vi "Update Enum Value.vi"(9 "Value":string, 10 "Tree Tag":string, 11 "UI Data In":refnum<class "Settings UI.lvclass">) -> (3 "UI Data Out":refnum<class "Settings UI.lvclass">)   [LabVIEW 2024, in "Output Sequencer.lvlib" / "Settings UI.lvclass"]
uses:
  Settings UI.lvclass
  Settings UI.lvclass/Settings UI.ctl
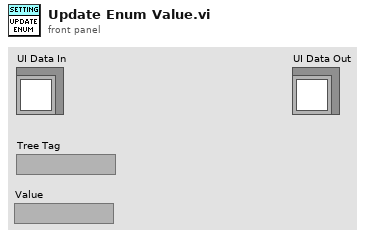
[diagram p1: front panel]
types:
  T1 = typedef "Output Sequencer.lvlib/Settings UI.lvclass/Tree Index Enum.ctl" = enum16{"General Settings", "Num Steps", "Num Analog", "Num Digital", "Show Confirmation", "Interp Priority", "Adv Timing", "Enable Conditions", "Seq Execution", "Reset Test Start", "Only When Test", "Delay After Test", "Start condition", "Re-triggering", "Stop condition", "Stop After Cycles", "Stop Values", "Default Values", "Default Analog", "Default Digital", "Steps", "Step #", "Description", "Precondition", "Duration", "Mode", "Delay Between Vals", "Analog Values", "Digital Values", "Postcondition", "On True", "On False"}
  T2 = typedef "Output Sequencer.lvlib/Settings UI.lvclass/Tree Item Settings.ctl" = cluster{"Tree Label":string, "Indent Level":i32, "Data Type":T3, "Numeric Range":cluster{"Min":dbl, "Max":dbl, "Inc":dbl}, "Allowed Values":string[], "Default Value":string, "Description":string}
  T3 = typedef "Output Sequencer.lvlib/Settings UI.lvclass/Data Type.ctl" = i16
  T4 = typedef "Output Sequencer.lvlib/Settings UI.lvclass/Step Settings.ctl" = cluster{"Description":string, "Precondition":string, "Duration":dbl, "Mode":string, "Delay Between Values":dbl, "Analog Values":string[], "Digital Values":string[], "Postcondition":string, "On True":string, "On False":string}
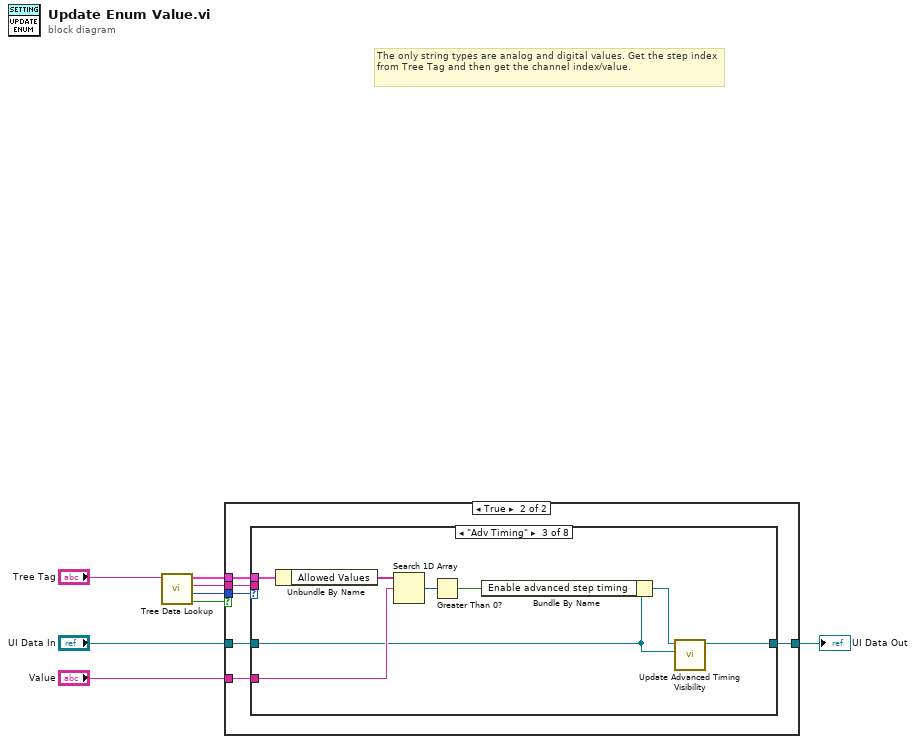
[diagram p0: block diagram]
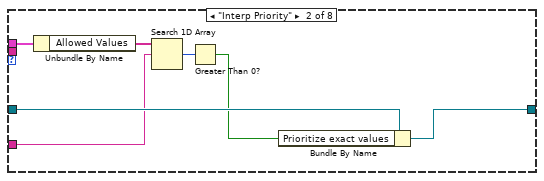
[diagram p4: hidden frame]
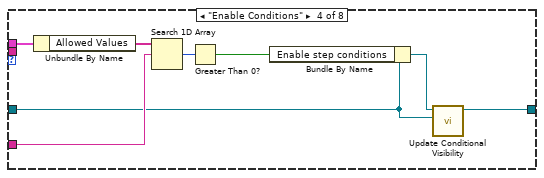
[diagram p5: hidden frame]
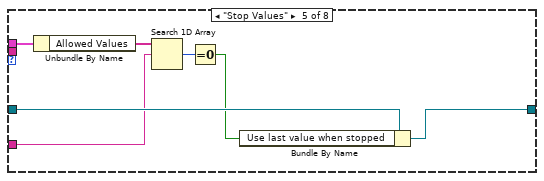
[diagram p6: hidden frame]
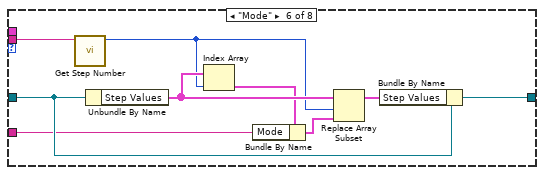
[diagram p7: hidden frame]
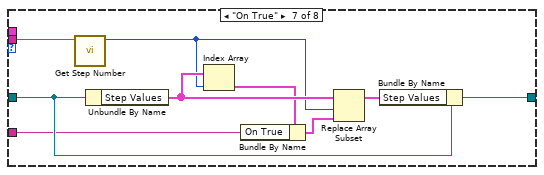
[diagram p8: hidden frame]
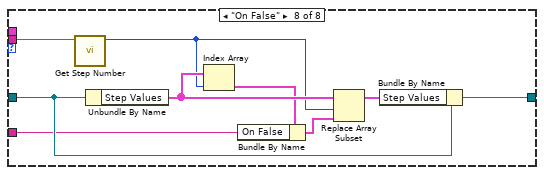
[diagram p9: hidden frame]
diagram:
  # "The only string types are analog and digital values. Get the step index from Tree Tag and then get the channel index/value."
  n1 = call "Tree Data Lookup.vi"("Tag in"="Tree Tag") -> ("Found?"=w4:bool, "Tree Index Enum"=w3:T1, "Tag out"=w1:string, "Tree Data"=w2:T2)  [unwired: 5 in, 2 out]
  n2 = case shown="True" w4 {
    tunnel: "UI Data In" -> [w9 w15]
    tunnel: [w9 w14] -> w7
    tunnel: "Value" -> [_ w13]
    tunnel: w3 -> [_ w12]
    tunnel: w2 -> [_ w11]
    tunnel: w1 -> [_ w10]
    frame False {
    }
    frame True {
      n3 = case shown="\"Adv Timing\"" w12 {
        tunnel: w15 -> [w16 w23 w27 w35 w46 w51 w60 w69]
        tunnel: [w16 w18 w24 w32 w41 w50 w59 w68] -> w14
        tunnel: w13 -> [_ w21 w30 w38 w44 w49 w58 w67]
        tunnel: w11 -> [_ w17 w26 w34 w40 _ _ _]
        tunnel: w10 -> [_ _ _ _ _ w48 w57 w66]
        frame Default {
        }
        frame "Interp Priority" {
          n4 = Unbundle By Name(w17) -> ("Allowed Values"=w22:string[])
          n5 = Search 1D Array(1D array=w22, element=w21) -> (index of element=w20:i32)  [unwired: 1 in]
          n6 = Greater Than 0?(x=w20) -> (x > 0?=w19:bool)
          n7 = Bundle By Name(cluster=w23, "Prioritize exact values"=w19) -> (w18:refnum<class "Settings UI.lvclass">)
        }
        frame "Adv Timing" {
          n8 = Unbundle By Name(w26) -> ("Allowed Values"=w31:string[])
          n9 = Search 1D Array(1D array=w31, element=w30) -> (index of element=w29:i32)  [unwired: 1 in]
          n10 = Greater Than 0?(x=w29) -> (x > 0?=w28:bool)
          n11 = Bundle By Name(cluster=w27, "Enable advanced step timing"=w28) -> (w25:refnum<class "Settings UI.lvclass">)
          n12 = call "Update Advanced Timing Visibility.vi"("Previous UI Data in"=w27, "New UI Data in"=w25) -> ("New UI Data out"=w24:refnum<class "Settings UI.lvclass">)  [unwired: 8 in, 1 out]
        }
        frame "Enable Conditions" {
          n13 = Unbundle By Name(w34) -> ("Allowed Values"=w39:string[])
          n14 = Search 1D Array(1D array=w39, element=w38) -> (index of element=w37:i32)  [unwired: 1 in]
          n15 = Greater Than 0?(x=w37) -> (x > 0?=w36:bool)
          n16 = Bundle By Name(cluster=w35, "Enable step conditions"=w36) -> (w33:refnum<class "Settings UI.lvclass">)
          n17 = call "Update Conditional Visibility.vi"("Previous UI Data in"=w35, "New UI Data in"=w33) -> ("New UI Data out"=w32:refnum<class "Settings UI.lvclass">)  [unwired: 9 in]
        }
        frame "Stop Values" {
          n18 = Unbundle By Name(w40) -> ("Allowed Values"=w45:string[])
          n19 = Search 1D Array(1D array=w45, element=w44) -> (index of element=w43:i32)  [unwired: 1 in]
          n20 = Equal To 0?(x=w43) -> (x = 0?=w42:bool)
          n21 = Bundle By Name(cluster=w46, "Use last value when stopped"=w42) -> (w41:refnum<class "Settings UI.lvclass">)
        }
        frame "Mode" {
          n22 = call "Get Step Number.vi"("Tree Tag"=w48) -> ("Step Number"=w47:i32)  [unwired: 8 in, 2 out]
          n23 = Unbundle By Name(w51) -> ("Step Values"=w55:T4[])
          n24 = Index Array(array=w55, index=w47) -> (element=w53:T4)
          n25 = Bundle By Name(cluster=w53, "Mode"=w49) -> (w52:T4)
          n26 = Replace Array Subset(array=w55, new element=w52, index=w47) -> (w54:T4[])
          n27 = Bundle By Name(cluster=w51, "Step Values"=w54) -> (w50:refnum<class "Settings UI.lvclass">)
        }
        frame "On True" {
          n28 = call "Get Step Number.vi"("Tree Tag"=w57) -> ("Step Number"=w56:i32)  [unwired: 8 in, 2 out]
          n29 = Unbundle By Name(w60) -> ("Step Values"=w64:T4[])
          n30 = Index Array(array=w64, index=w56) -> (element=w62:T4)
          n31 = Bundle By Name(cluster=w62, "On True"=w58) -> (w61:T4)
          n32 = Replace Array Subset(array=w64, new element=w61, index=w56) -> (w63:T4[])
          n33 = Bundle By Name(cluster=w60, "Step Values"=w63) -> (w59:refnum<class "Settings UI.lvclass">)
        }
        frame "On False" {
          n34 = call "Get Step Number.vi"("Tree Tag"=w66) -> ("Step Number"=w65:i32)  [unwired: 8 in, 2 out]
          n35 = Unbundle By Name(w69) -> ("Step Values"=w73:T4[])
          n36 = Index Array(array=w73, index=w65) -> (element=w71:T4)
          n37 = Bundle By Name(cluster=w71, "On False"=w67) -> (w70:T4)
          n38 = Replace Array Subset(array=w73, new element=w70, index=w65) -> (w72:T4[])
          n39 = Bundle By Name(cluster=w69, "Step Values"=w72) -> (w68:refnum<class "Settings UI.lvclass">)
        }
      }
    }
  }
  "UI Data Out" <- w7
